vi "isOpen.vi"(8 "error in (no error)":errorcluster, 11 "CCD in":refnum<class "CCD.lvclass">) -> (0 "error out":errorcluster, 2 "CCD is open?":T1, 3 "CCD out":refnum<class "CCD.lvclass">)   [LabVIEW 2023, in "CCD.lvclass"]
uses:
  CCD.lvclass
  ccdIsOpen.ctl
  d9b87029-586e-44ee-a6e5-d4a5e0edce38.vi
  b59fd1e7-dcda-425c-bd6c-61aafb79e7f4.vi
  <vilib>/JDP Science/JSONtext/Variant to JSON Text.vi
  <vilib>/JDP Science/JSONtext/Set Item.vi
  <vilib>/JDP Science/JSONtext/JSON text to Variant.vi
  <vilib>/JDP Science/JSONtext/LVClass Serializer/JSONtext LVClass Serializer.lvclass
  CCD.lvclass/CCD.ctl
  GenericDevice/GenericDevice.lvclass
panel:
  # "Connector Pane"
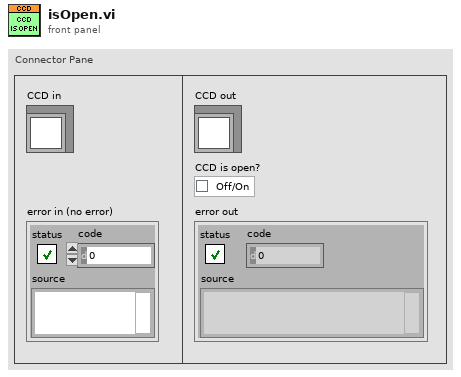
[diagram p1: front panel]
types:
  T1 = typedef "CCD.lvclass/ccdIsOpen.ctl" = cluster{"Checkbox":bool}
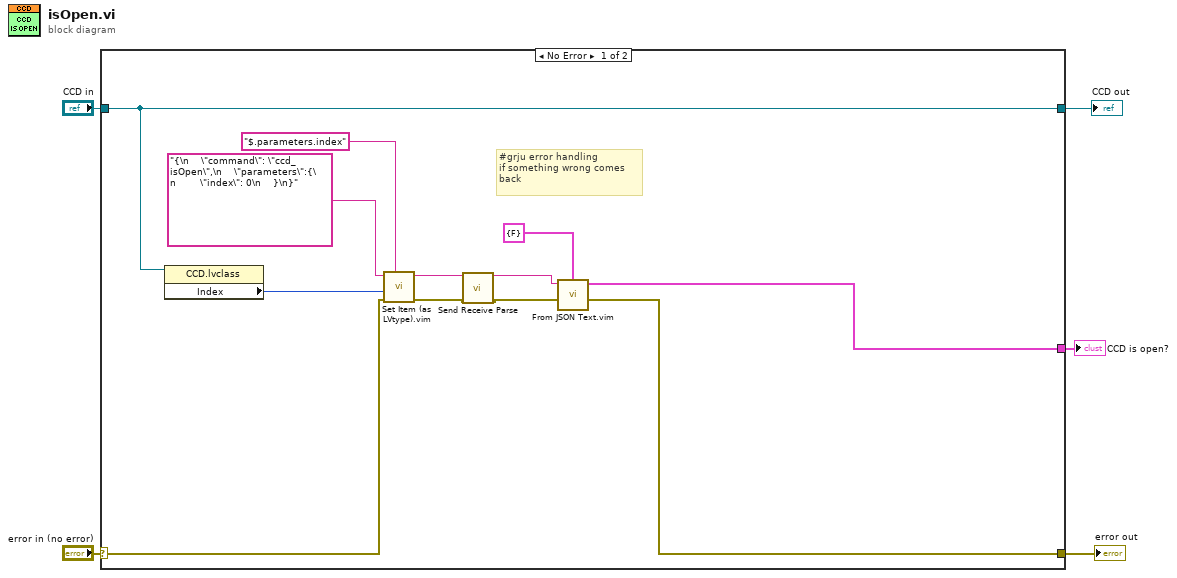
[diagram p0: block diagram]
diagram:
  n1 = case shown="No Error" "error in (no error)" {
    selector: "error in (no error)" -> [w13 w19]
    tunnel: [w11 w19] -> w4
    tunnel: [w15 w18] -> w2
    tunnel: "CCD in" -> [w15 w18]
    tunnel: [w12 _] -> w1
    frame No Error {
      # "#grju error handling\nif something wrong comes\nback"
      n2 = property class="CCD.lvclass"(reference=w15) -> ("Index"=w14:i32)  [unwired: 1 in, 2 out]
      n3 = call "Set Item (as LVtype).vim"("$Path or Item Name"="$.parameters.index", "error in (no error)"=w13, "Anything"=w14, "JSON"="{\n    \"command\": \"ccd_isOpen\",\n    \"parameters\":{\n        \"index\": 0\n    }\n}") -> ("error out"=w8:errorcluster, "<JSON>"=w9:string)  [unwired: 4 in, 1 out]
      n4 = call "Send Receive Parse.vi"("<JSON>"=w9, "error in"=w8) -> ("results-JSON string"=w7:string, "error out"=w6:errorcluster)  [unwired: 9 in, 7 out]
      n5 = call "From JSON Text.vim"("Data Type and Default Value"=T1 {"Checkbox"=FALSE} ("Cluster"), "error in (no error)"=w6, "JSON"=w7) -> ("error out"=w11:errorcluster, "Data out"=w12:T1)  [unwired: 7 in]
    }
    frame Error {
    }
  }
  "error out" <- w4
  "CCD out" <- w2
  "CCD is open?" <- w1
